vi "ReadDB.vi"() -> ()   [LabVIEW 2018]
uses:
  <vilib>/addons/database/Connection.llb/DB Tools Open Connec (Path).vi
  <vilib>/addons/database/_DB Variant To Data/Database Variant To Data.xnode
  <vilib>/addons/database/NI_Database_API.lvlib
panel:
  out "数组":T1(array[cluster])
  out "条目数":i32
  out "error out":errorcluster {"code" format="%x"}
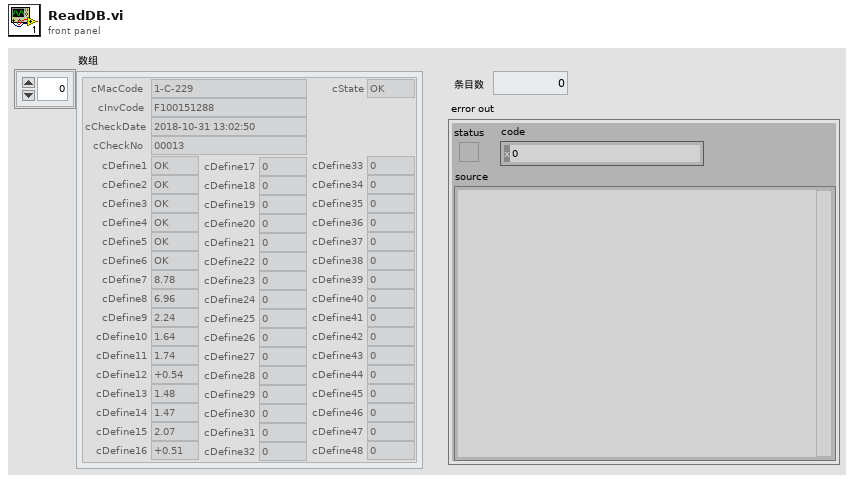
[diagram p1: front panel]
types:
  T1 = cluster{"cMacCode":string, "cInvCode":string, "cCheckDate":string, "cCheckNo":string, "cState":string, "cDefine1":string, "cDefine2":string, "cDefine3":string, "cDefine4":string, "cDefine5":string, "cDefine6":string, "cDefine7":string, "cDefine8":string, "cDefine9":string, "cDefine10":string, "cDefine11":string, "cDefine12":string, "cDefine13":string, "cDefine14":string, "cDefine15":string, "cDefine16":string, "cDefine17":string, "cDefine18":string, "cDefine20":string, "cDefine19":string, "cDefine21":string, "cDefine22":string, "cDefine23":string, "cDefine24":string, "cDefine25":string, "cDefine26":string, "cDefine27":string, "cDefine28":string, "cDefine29":string, "cDefine30":string, "cDefine31":string, "cDefine32":string, "cDefine33":string, "cDefine34":string, "cDefine35":string, "cDefine36":string, "cDefine37":string, "cDefine38":string, "cDefine39":string, "cDefine40":string, "cDefine41":string, "cDefine42":string, "cDefine43":string, "cDefine44":string, "cDefine45":string, "cDefine46":string, "cDefine47":string, "cDefine48":string}[]
  T2 = typedef "NI_Database_API.lvlib/Conn ObjectReference.ctl" = refnum<k1>
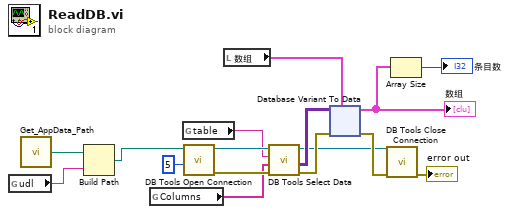
[diagram p0: block diagram]
diagram:
  n1 = global read "全局SQL.vi" "udl"() -> (w1:string)
  n2 = call "Get_AppData_Path.vi"() -> ("path"=w15:path)  [unwired: 1 in]
  n3 = Build Path(base path=w15, name or relative path=w1) -> (appended path=w14:path)
  n4 = global read "全局SQL.vi" "Columns"() -> (w3:string[])
  n5 = global read "全局SQL.vi" "table"() -> (w2:string)
  n6 = call-poly <vilib>:"DB Tools Open Connection.vi"("connection timeout (15)"=5, "connection information"=w14) -> ("error out"=w11:errorcluster, "connection reference"=w12:T2)  [unwired: 6 in]
  n7 = local read "数组"() -> (w4:T1)
  n8 = call <vilib>:"DB Tools Select Data.vi"("error in (no error)"=w11, "columns"=w3, "table"=w2, "connection reference"=w12) -> ("error out"=w10:errorcluster, "data"=w8:variant[][], "connection reference out"=w7:T2)  [unwired: 2 in]
  n9 = xnode "Database Variant To Data"("database variant"=w8, "error in (no error)"=w10, "type"=w4) -> ("data"=w5:T1, "error out"=w9:errorcluster)
  "数组" <- w5
  n10 = call <vilib>:"DB Tools Close Connection.vi"("error in (no error)"=w9, "connection reference"=w7) -> ("error out"=→"error out":errorcluster)  [unwired: 5 in]
  n11 = Array Size(array=w5) -> (size(s)=→"条目数":i32)
